vi "GetDeviceEquipmentProperties.vi"(10 "equipment Ids":string[](array[string]), 11 "equipment list":T2[](array[typedef])) -> (2 "tdms properties":T1[](array[typedef]))   [LabVIEW 2017, in "Tdms.lvlib"]
doc: "Returns TDMS properties that define the names of nodes in the NI InsightCM Server equipment layout to which a data group is assigned. Use the TDMS Set Properties function to write these properties to a TDMS file that contains data from the channels in the data group."
uses:
  <vilib>/addons/InsightCM/Utilities/Tdms/Tdms.lvlib
  <vilib>/addons/InsightCM/MessageBus/Base/controls/Equipment.ctl
  <vilib>/addons/InsightCM/MessageBus/Base/controls/KeyValuePair.ctl
  <vilib>/addons/InsightCM/Utilities/Tdms/controls/Property.ctl
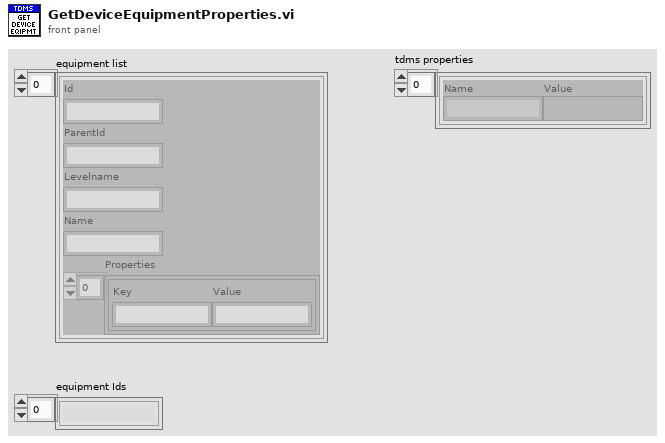
[diagram p1: front panel]
types:
  T1 = typedef "Tdms.lvlib/Property.ctl" = cluster{"Name":string, "Value":variant}
  T2 = typedef "Equipment.ctl" = cluster{"Id":string, "ParentId":string, "Levelname":string, "Name":string, "Properties":T3[]}
  T3 = typedef "KeyValuePair.ctl" = cluster{"Key":string, "Value":string}
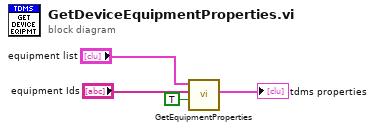
[diagram p0: block diagram]
diagram:
  n1 = call <vilib>:"GetEquipmentProperties.vi"("Device"=TRUE, "EquipmentIds"="equipment Ids", "Equipment List"="equipment list") -> ("Tdms Properties"=→"tdms properties":T1[])  [unwired: 8 in]
